vi "0036-Sub_graph.vi"(7 "温湿度データ":dbl[][](array[numeric])) -> (1 "温度":T1, 3 "湿度":T1)   [LabVIEW 2014]
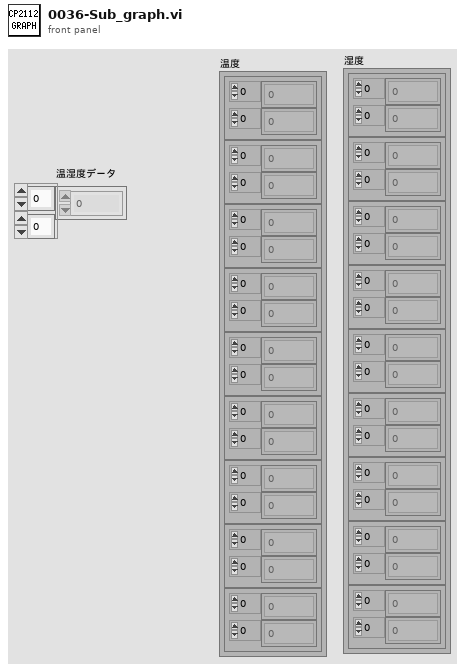
[diagram p1: front panel]
types:
  T1 = cluster{cluster{dbl[], dbl[]}, cluster{dbl[], dbl[]}, cluster{dbl[], dbl[]}, cluster{dbl[], dbl[]}, cluster{dbl[], dbl[]}, cluster{dbl[], dbl[]}, cluster{dbl[], dbl[]}, cluster{dbl[], dbl[]}, cluster{dbl[], dbl[]}}
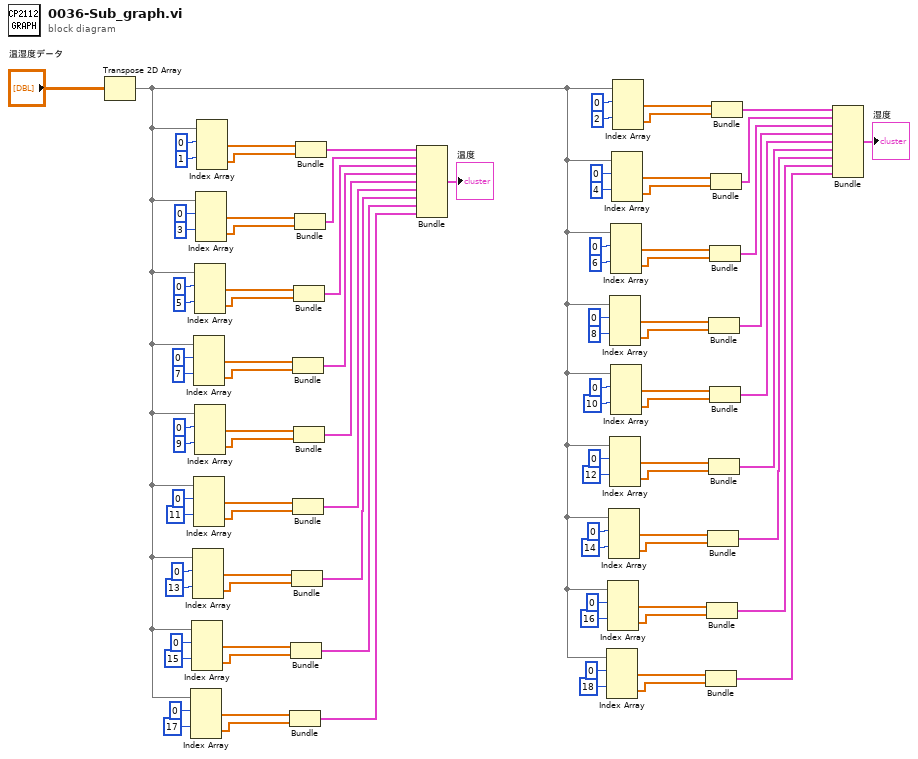
[diagram p0: block diagram]
diagram:
  n1 = Transpose 2D Array(2D array="温湿度データ") -> (transposed array=w1:dbl[][])
  n2 = Index Array(array=w1, index (row) #1=0 ("指標 （行）"), index (row) #2=17 ("指標 （行）")) -> (element #1=w57:dbl[], element #2=w56:dbl[])  [unwired: 2 in]
  n3 = Index Array(array=w1, index (row) #1=0 ("指標 （行）"), index (row) #2=15 ("指標 （行）")) -> (element #1=w61:dbl[], element #2=w60:dbl[])  [unwired: 2 in]
  n4 = Index Array(array=w1, index (row) #1=0 ("指標 （行）"), index (row) #2=13 ("指標 （行）")) -> (element #1=w65:dbl[], element #2=w64:dbl[])  [unwired: 2 in]
  n5 = Index Array(array=w1, index (row) #1=0 ("指標 （行）"), index (row) #2=7 ("指標 （行）")) -> (element #1=w77:dbl[], element #2=w76:dbl[])  [unwired: 2 in]
  n6 = Index Array(array=w1, index (row) #1=0 ("指標 （行）"), index (row) #2=11 ("指標 （行）")) -> (element #1=w69:dbl[], element #2=w68:dbl[])  [unwired: 2 in]
  n7 = Index Array(array=w1, index (row) #1=0 ("指標 （行）"), index (row) #2=5 ("指標 （行）")) -> (element #1=w81:dbl[], element #2=w80:dbl[])  [unwired: 2 in]
  n8 = Index Array(array=w1, index (row) #1=0 ("指標 （行）"), index (row) #2=9 ("指標 （行）")) -> (element #1=w73:dbl[], element #2=w72:dbl[])  [unwired: 2 in]
  n9 = Index Array(array=w1, index (row) #1=0 ("指標 （行）"), index (row) #2=3 ("指標 （行）")) -> (element #1=w87:dbl[], element #2=w86:dbl[])  [unwired: 2 in]
  n10 = Index Array(array=w1, index (row) #1=0 ("指標 （行）"), index (row) #2=1 ("指標 （行）")) -> (element #1=w91:dbl[], element #2=w90:dbl[])  [unwired: 2 in]
  n11 = Bundle(w57, w56) -> (w49:cluster{dbl[], dbl[]})  [unwired: 1 in]
  n12 = Bundle(w61, w60) -> (w50:cluster{dbl[], dbl[]})  [unwired: 1 in]
  n13 = Bundle(w65, w64) -> (w51:cluster{dbl[], dbl[]})  [unwired: 1 in]
  n14 = Bundle(w77, w76) -> (w54:cluster{dbl[], dbl[]})  [unwired: 1 in]
  n15 = Bundle(w69, w68) -> (w52:cluster{dbl[], dbl[]})  [unwired: 1 in]
  n16 = Bundle(w81, w80) -> (w55:cluster{dbl[], dbl[]})  [unwired: 1 in]
  n17 = Bundle(w73, w72) -> (w53:cluster{dbl[], dbl[]})  [unwired: 1 in]
  n18 = Bundle(w87, w86) -> (w84:cluster{dbl[], dbl[]})  [unwired: 1 in]
  n19 = Bundle(w91, w90) -> (w85:cluster{dbl[], dbl[]})  [unwired: 1 in]
  n20 = Bundle(w85, w84, w55, w54, w53, w52, w51, w50, w49) -> (→"温度":T1)  [unwired: 1 in]
  n21 = Index Array(array=w1, index (row) #1=0 ("指標 （行）"), index (row) #2=18 ("指標 （行）")) -> (element #1=w11:dbl[], element #2=w10:dbl[])  [unwired: 2 in]
  n22 = Index Array(array=w1, index (row) #1=0 ("指標 （行）"), index (row) #2=16 ("指標 （行）")) -> (element #1=w15:dbl[], element #2=w14:dbl[])  [unwired: 2 in]
  n23 = Index Array(array=w1, index (row) #1=0 ("指標 （行）"), index (row) #2=14 ("指標 （行）")) -> (element #1=w19:dbl[], element #2=w18:dbl[])  [unwired: 2 in]
  n24 = Index Array(array=w1, index (row) #1=0 ("指標 （行）"), index (row) #2=8 ("指標 （行）")) -> (element #1=w31:dbl[], element #2=w30:dbl[])  [unwired: 2 in]
  n25 = Index Array(array=w1, index (row) #1=0 ("指標 （行）"), index (row) #2=12 ("指標 （行）")) -> (element #1=w23:dbl[], element #2=w22:dbl[])  [unwired: 2 in]
  n26 = Index Array(array=w1, index (row) #1=0 ("指標 （行）"), index (row) #2=6 ("指標 （行）")) -> (element #1=w35:dbl[], element #2=w34:dbl[])  [unwired: 2 in]
  n27 = Index Array(array=w1, index (row) #1=0 ("指標 （行）"), index (row) #2=10 ("指標 （行）")) -> (element #1=w27:dbl[], element #2=w26:dbl[])  [unwired: 2 in]
  n28 = Index Array(array=w1, index (row) #1=0 ("指標 （行）"), index (row) #2=4 ("指標 （行）")) -> (element #1=w41:dbl[], element #2=w40:dbl[])  [unwired: 2 in]
  n29 = Index Array(array=w1, index (row) #1=0 ("指標 （行）"), index (row) #2=2 ("指標 （行）")) -> (element #1=w45:dbl[], element #2=w44:dbl[])  [unwired: 2 in]
  n30 = Bundle(w11, w10) -> (w3:cluster{dbl[], dbl[]})  [unwired: 1 in]
  n31 = Bundle(w15, w14) -> (w4:cluster{dbl[], dbl[]})  [unwired: 1 in]
  n32 = Bundle(w19, w18) -> (w5:cluster{dbl[], dbl[]})  [unwired: 1 in]
  n33 = Bundle(w31, w30) -> (w8:cluster{dbl[], dbl[]})  [unwired: 1 in]
  n34 = Bundle(w23, w22) -> (w6:cluster{dbl[], dbl[]})  [unwired: 1 in]
  n35 = Bundle(w35, w34) -> (w9:cluster{dbl[], dbl[]})  [unwired: 1 in]
  n36 = Bundle(w27, w26) -> (w7:cluster{dbl[], dbl[]})  [unwired: 1 in]
  n37 = Bundle(w41, w40) -> (w38:cluster{dbl[], dbl[]})  [unwired: 1 in]
  n38 = Bundle(w45, w44) -> (w39:cluster{dbl[], dbl[]})  [unwired: 1 in]
  n39 = Bundle(w39, w38, w9, w8, w7, w6, w5, w4, w3) -> (→"湿度":T1)  [unwired: 1 in]
